vi "ALTS-2015 OPC engine initialize.vi"(8 "error in (no error)":errorcluster, 9 "ms timeout (10000)":i32=10000, 10 "mode":T1(ring), 11 "URLs":string[](array[string])) -> (0 "error out":errorcluster, 3 "Connection ids":refnum<k13>[](array[refnum]))   [LabVIEW 2013]
doc: "Copyright © 2005, Soliton Technologies.\nAll rights reserved."
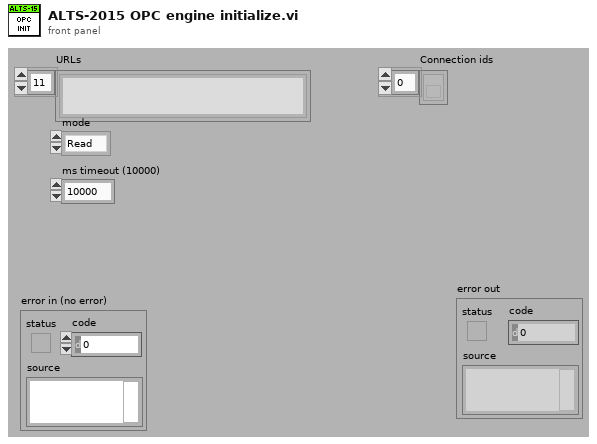
[diagram p1: front panel]
types:
  T1 = enum16{"Read", "Write", "ReadWrite", "BufferedRead", "BufferedReadWrite"}
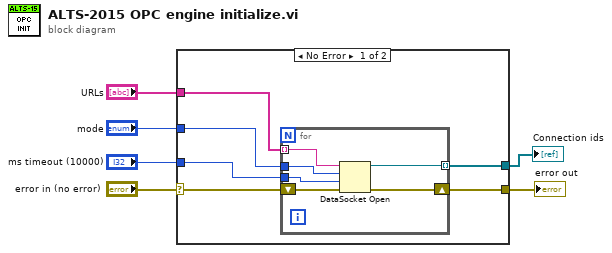
[diagram p0: block diagram]
diagram:
  n1 = case shown="No Error" "error in (no error)" {
    selector: "error in (no error)" -> [w11 w20]
    tunnel: [w10 w20] -> w5
    tunnel: "URLs" -> [w12 _]
    tunnel: "mode" -> [w9 _]
    tunnel: "ms timeout (10000)" -> [w8 _]
    tunnel: [w7 refnum<k13>[] []] -> w1
    frame No Error {
      n2 = for {
        tunnel: w12 -> [w18] mode=indexing
        shift-right: [w16] -> w10
        shift-left: w11 -> [w17]
        tunnel: w9 -> [w15]
        tunnel: w8 -> [w14]
        tunnel: [w13] -> w7 mode=indexing
        n3 = DataSocket Open(8:w17, 9:w14, 10:w15, 11:w18) -> (0:w16:errorcluster, 3:w13:refnum<k13>)
      }
    }
    frame Error {
    }
  }
  "error out" <- w5
  "Connection ids" <- w1
